vi "Get Active Binding Post.vi"(8 "error in (no error)":errorcluster, 11 "VISA resource name":refnum<visa-resource-name>) -> (0 "error out":errorcluster, 2 "Current Output Post":i32, 3 "VISA resource name out":refnum<visa-resource-name>)   [LabVIEW 2014, in "Fluke 5XXX Series Multicalibrators.lvlib"]
doc: "This VI returns the binding posts for current output.\n\nNote:\n\nThis VI is available only for instrument models 5700A, 5720A and 57LFC."
uses:
  Fluke 5XXX Series Multicalibrators.lvlib
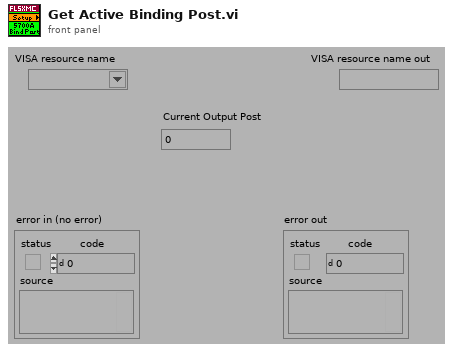
[diagram p1: front panel]
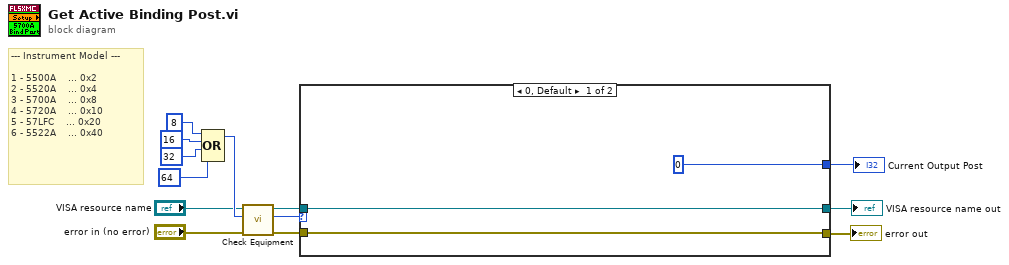
[diagram p0: block diagram]
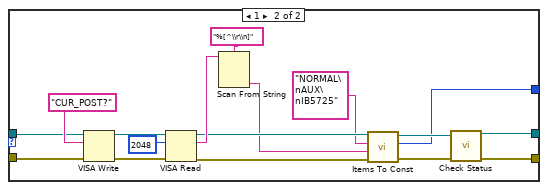
[diagram p2: hidden frame]
diagram:
  # "--- Instrument Model ---\n\n1 - 5500A    ... 0x2\n2 - 5520A    ... 0x4\n3 - 5700A    ... 0x8\n4 - 5720A    ... 0x10\n5 - 57LFC    ... 0x20\n6 - 5522A    ... 0x40"
  n1 = Compound Arithmetic op=OR(8 ("Numeric"), 16 ("Numeric"), 32 ("Numeric"), 64 ("Numeric")) -> (w8:i32)
  n2 = call "Check Equipment.vi"("error in (no error)"="error in (no error)", "Bit Mask"=w8, "VISA resource name"="VISA resource name") -> ("error out"=w13:errorcluster, "Present?"=w12:u32, "VISA resource name out"=w11:refnum<visa-resource-name>)  [unwired: 6 in]
  n3 = case shown="0, Default" w12 {
    tunnel: [w16 w27] -> w7
    tunnel: [w15 w26] -> w6
    tunnel: w13 -> [w16 w29]
    tunnel: w11 -> [w15 w28]
    tunnel: [0 w17] -> w3
    frame 0, Default {
    }
    frame 1 {
      n4 = VISA Write(VISA resource name=w28, write buffer="CUR_POST?", error in (no error)=w29) -> (VISA resource name out=w32:refnum<visa-resource-name>, error out=w31:errorcluster)  [unwired: 1 out]
      n5 = VISA Read(VISA resource name=w32, byte count=u32 2048 ("byte count (0)"), error in (no error)=w31) -> (VISA resource name out=w21:refnum<visa-resource-name>, read buffer=w24:string, error out=w22:errorcluster)  [unwired: 1 out]
      n6 = Scan From String(format string="%[^\\r\\n]", input string=w24) -> (output 1=w18:string)  [unwired: 3 in, 3 out]
      n7 = call "Items To Const.vi"("error in (no error)"=w22, "String Item"=w18, "Multi-Line String"="NORMAL\nAUX\nIB5725", "VISA resource name"=w21) -> ("error out"=w23:errorcluster, "Index"=w17:i32, "VISA resource name out"=w20:refnum<visa-resource-name>)  [unwired: 5 in]
      n8 = call "Check Status.vi"("VISA resource name"=w20, "error in (no error)"=w23) -> ("VISA resource name out"=w26:refnum<visa-resource-name>, "error out"=w27:errorcluster)  [unwired: 12 in]
    }
  }
  "Current Output Post" <- w3
  "VISA resource name out" <- w6
  "error out" <- w7
